vi ".NET Folder Dialog.vi"(7 "Dialog Message":string, 8 "Error In":errorcluster, 9 "Root Folder":i32(ring) items=["Desktop"=0, "Programs"=2, "MyDocuments, Personal"=5, "Favorites"=6, "Startup"=7, "Recent"=8, "SendTo"=9, "StartMenu"=11, "MyMusic"=13, "MyVideos"=14, "DesktopDirectory"=16, "MyComputer"=17, "NetworkShortcuts"=19, "Fonts"=20, "Templates"=21, "CommonStartMenu"=22, "CommonPrograms"=23, "CommonStartup"=24, "CommonDesktopDirectory"=25, "ApplicationData"=26, "PrinterShortcuts"=27, "LocalApplicationData"=28, "InternetCache"=32, "Cookies"=33, "History"=34, "CommonApplicationData"=35, "Windows"=36, "System"=37, "ProgramFiles"=38, "MyPictures"=39, "UserProfile"=40, "SystemX86"=41, "ProgramFilesX86"=42, "CommonProgramFiles"=43, "CommonProgramFilesX86"=44, "CommonTemplates"=45, "CommonDocuments"=46, "CommonAdminTools"=47, "AdminTools"=48, "CommonMusic"=53, "CommonPictures"=54, "CommonVideos"=55, "Resources"=56, "LocalizedResources"=57, "CommonOemLinks"=58, "CDBurning"=59], 10 "Show New Folder Button":bool=TRUE, 11 "Selected Path":path) -> (0 "Error Out":errorcluster, 1 "Cancelled?":bool, 3 "Selected Path":path)   [LabVIEW 2021, in "Files.lvlib"]
uses:
  System.Windows.Forms
  Files.lvlib
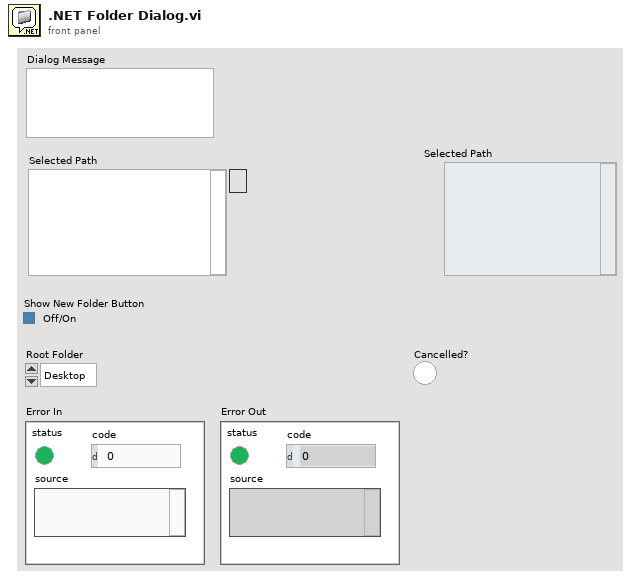
[diagram p1: front panel]
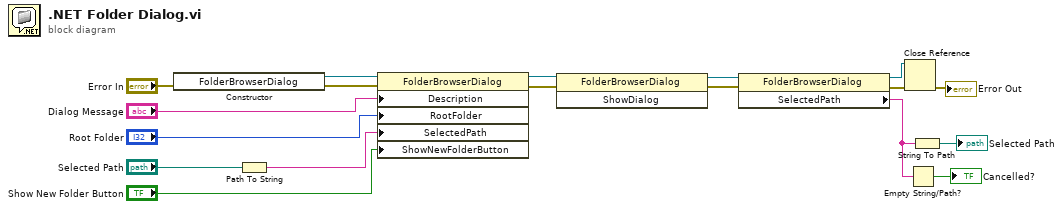
[diagram p0: block diagram]
diagram:
  n1 = constructor class="FolderBrowserDialog"(error in="Error In") -> (reference out=w18:refnum<k24>, error out=w17:errorcluster)  [unwired: 2 in, 1 out]
  n2 = Path To String(path="Selected Path") -> (string=w1:string)
  n3 = property class="FolderBrowserDialog"(reference=w18, error in=w17, "Description"="Dialog Message", "RootFolder"="Root Folder", "SelectedPath"=w1, "ShowNewFolderButton"="Show New Folder Button") -> (reference out=w14:refnum<k24>, error out=w13:errorcluster)
  n4 = invoke class="FolderBrowserDialog" method="ShowDialog"(reference=w14, error in=w13) -> (reference out=w12:refnum<k24>, error out=w11:errorcluster)  [unwired: 1 in, 1 out]
  n5 = property class="FolderBrowserDialog"(reference=w12, error in=w11) -> (reference out=w9:refnum<k24>, error out=w10:errorcluster, "SelectedPath"=w3:string)
  n6 = Close Reference(reference=w9, error in (no error)=w10) -> (error out=→"Error Out":errorcluster)
  n7 = Empty String/Path?(string/path=w3) -> (empty?=→"Cancelled?":bool)
  n8 = String To Path(string=w3) -> (path=→"Selected Path":path)
